vi "GOOP_LVClass_Item_NotifyChanged.vi"(10 "Change Type":T1=enum."Item Modified", 11 "Object":u64) -> ()   [LabVIEW 2016]
uses:
  <resource>/Framework/Providers/API/mxLvChangeType.ctl
  <resource>/Framework/Providers/Open_GDS/SubVIs/GOOP_ClassProviderClassType.ctl
  <resource>/Framework/Providers/Open_GDS/ClassProviders/Provider_BaseClassInterface/ClassWriter_class/ClassWriter.lvclass
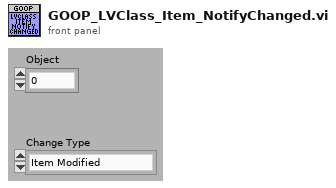
[diagram p1: front panel]
types:
  T1 = typedef "mxLvChangeType.ctl" = enum32{"Item Created", "Item Modified", "File Modified", "File Deleted", "Item Added", "Item Added to SCC", "Item Renamed", "Item Modified For SCC"}
  T2 = typedef "GOOP_ClassProviderClassType.ctl" = enum16{"ClassWriter", "ClassReader"}
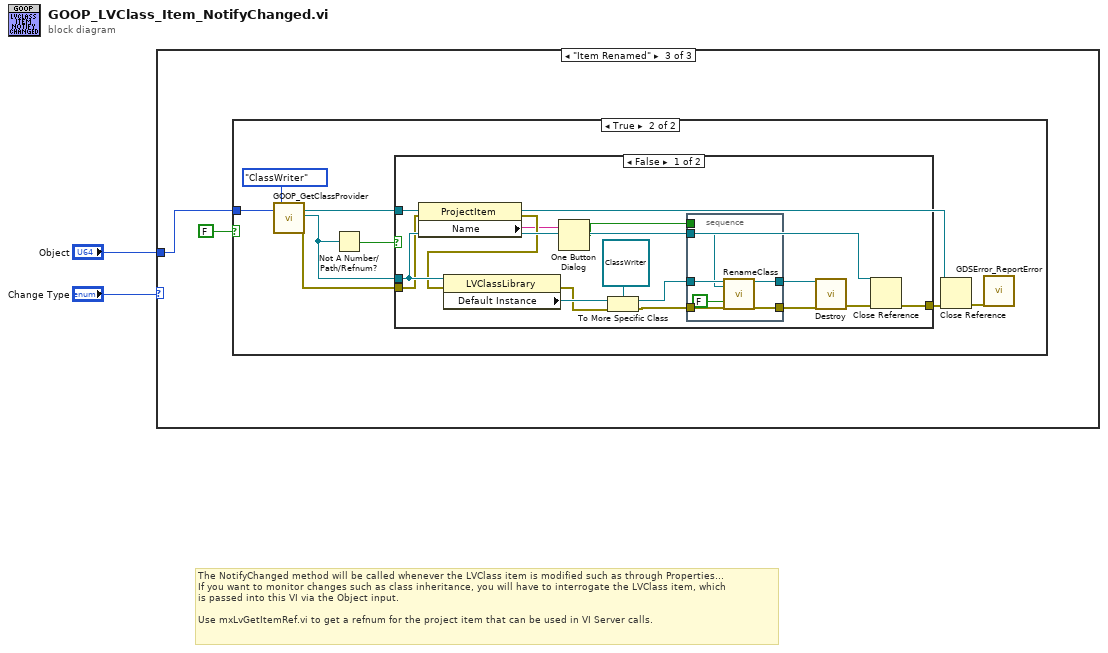
[diagram p0: block diagram]
diagram:
  # "The NotifyChanged method will be called whenever the LVClass item is modified such as through Properties...\nIf you want to monitor changes such as class inheritance, you will have to interrogate the LVClass item, which\nis passed into this VI via the Object input.\n\nUse mxLvGetItemRef.vi to get a refnum for the project item that can be used in VI Server calls."
  n1 = case shown="\"Item Renamed\"" "Change Type" {
    tunnel: "Object" -> [_ _ w4]
    frame "Item Created", Default {
    }
    frame "Item Modified" {
    }
    frame "Item Renamed" {
      n2 = case shown="True" FALSE {
        tunnel: w4 -> [_ w9]
        frame False {
        }
        frame True {
          n3 = call <resource>:"GOOP_GetClassProvider.vi"("New Item Parent/Object"=w9, "ProviderClassType"=GOOP_ClassProviderClassType."ClassWriter") -> ("ProjectItem"=w6:refnum<vi>, "LVClass.Open"=w8:refnum<vi>, "error out"=w12:errorcluster)  [unwired: 15 in]
          n4 = Not A Number/Path/Refnum?(number/path/refnum=w8) -> (NaN/Path/Refnum?=w7:bool)
          n5 = case shown="False" w7 {
            tunnel: w12 -> [w16 w34]
            tunnel: [w23 w34] -> w11
            tunnel: w8 -> [w18 _]
            tunnel: w6 -> [w17 _]
            frame False {
              n6 = property class="ProjectItem"(reference=w17, error in=w16) -> (error out=w15:errorcluster, "Name"=w14:string)  [unwired: 1 out]
              n7 = property class="LVClassLibrary"(reference=w18, error in=w15) -> (error out=w25:errorcluster, "Default Instance"=w27:refnum<class>)  [unwired: 1 out]
              n8 = One Button Dialog(message=w14) -> (true=w13:bool)  [unwired: 1 in]
              n9 = To More Specific Class(target class=refnum<class "ClassWriter.lvclass"> refnum ("ClassWriter.lvclass"), reference=w27, error in=w25) -> (specific class reference=w20:refnum<class "ClassWriter.lvclass">, error out=w19:errorcluster)
              n10 = stacked-sequence {
                tunnel: [w33] -> w22
                tunnel: [w32] -> w21
                tunnel: w20 -> [w31]
                tunnel: w19 -> [w30]
                tunnel: w18 -> [w29]
                tunnel: w13 -> [_]
                frame #0 {
                  n11 = call-dynamic "RenameClass.vi"("ClassWriter.lvclass"=w31, "ClassRef"=w29, "RelinkWholeProject"=FALSE, "error in (no error)"=w30) -> ("ClassWriter.lvclass"=w33:refnum<class "ClassWriter.lvclass">, "error out"=w32:errorcluster)  [unwired: 14 in]
                }
              }
              n12 = call-dynamic "Destroy.vi"("ClassWriter.lvclass"=w22, "error in (no error)"=w21) -> ("error out"=w24:errorcluster)  [unwired: 17 in]
              n13 = Close Reference(reference=w18, error in (no error)=w24) -> (error out=w23:errorcluster)
            }
            frame True {
            }
          }
          n14 = Close Reference(reference=w6, error in (no error)=w11) -> (error out=w5:errorcluster)
          n15 = call <resource>:"GDSError_ReportError.vi"("error in (no error)"=w5) -> ()  [unwired: 18 in, 1 out]
        }
      }
    }
  }
